vi "HW_6p1_Task2_pipoat.vi"() -> ()   [LabVIEW 2016]
panel:
  out "Verification (Percentage of above 250 C)":dbl
  out "Avg. Temp":dbl
  out "# Exceeding 250 degrees C":dbl
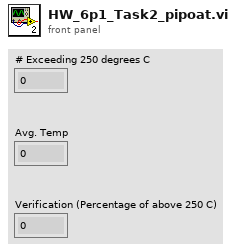
[diagram p1: front panel]
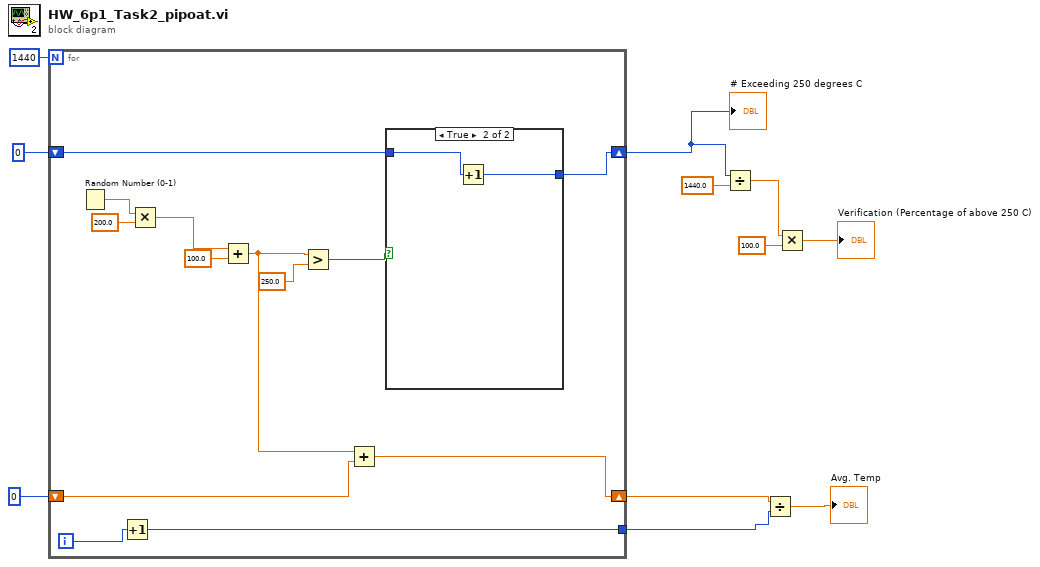
[diagram p0: block diagram]
diagram:
  n1 = for {
    N: 1440 -> [_]
    shift-right: [w13] -> w2
    shift-left: 0 -> [w20]
    shift-right: [w15] -> w6
    shift-left: 0 -> [w16]
    tunnel: [w12] -> w7
    i -> [w14]
    n2 = Random Number (0-1)() -> (number: 0 to 1=w24:dbl)
    n3 = Increment(x=w14) -> (x+1=w12:i32)
    n4 = Multiply(x=w24, y=200.0) -> (x*y=w22:dbl)
    n5 = Add(x=w22, y=100.0) -> (x+y=w17:dbl)
    n6 = Greater?(x=w17, y=250.0) -> (0:w18:bool)
    n7 = Add(x=w17, y=w16) -> (x+y=w15:dbl)
    n8 = case shown="True" w18 {
      tunnel: w20 -> [w25 w27]
      tunnel: [w25 w26] -> w13
      frame False {
      }
      frame True {
        n9 = Increment(x=w27) -> (x+1=w26:i32)
      }
    }
  }
  "# Exceeding 250 degrees C" <- w2
  n10 = Divide(x=w2, y=1440.0) -> (x/y=w1:dbl)
  n11 = Divide(x=w6, y=w7) -> (x/y=→"Avg. Temp":dbl)
  n12 = Multiply(x=w1, y=100.0) -> (x*y=→"Verification (Percentage of above 250 C)":dbl)
